vi "MatlabfileReader.vi"(8 "error in (no error)":errorcluster, 11 "Positions file":path) -> (0 "error out":errorcluster, 1 "Focus":dbl[](array[numeric]), 2 "Y":dbl[](array[numeric]), 3 "X":dbl[](array[numeric]), 5 "Time":dbl[](array[numeric]))   [LabVIEW 2012]
uses:
  <vilib>/Utility/file.llb/Read From Spreadsheet File (DBL).vi
  <vilib>/Analysis/NI_AALBase.lvlib
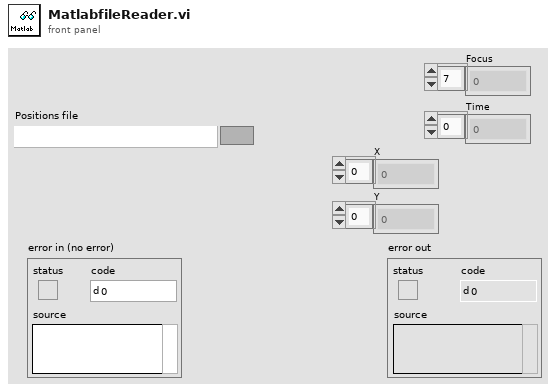
[diagram p1: front panel]
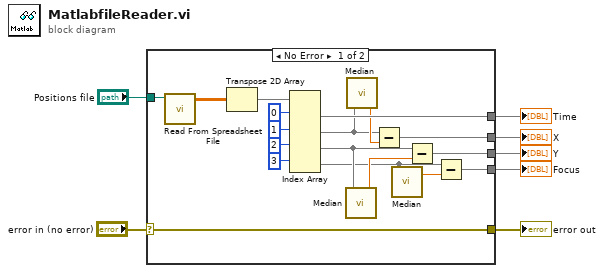
[diagram p0: block diagram]
diagram:
  n1 = case shown="No Error" "error in (no error)" {
    selector: "error in (no error)" -> [w20 w26]
    tunnel: [w20 w26] -> w6
    tunnel: "Positions file" -> [w25 _]
    tunnel: [w21 _] -> w4
    tunnel: [w14 _] -> w2
    tunnel: [w12 _] -> w3
    tunnel: [w13 _] -> w1
    frame No Error {
      n2 = call-poly <vilib>:"Read From Spreadsheet File.vi"("file path (dialog if empty)"=w25) -> ("all rows"=w24:dbl[][])  [unwired: 6 in, 4 out]
      n3 = Transpose 2D Array(2D array=w24) -> (transposed array=w19:dbl[][])
      n4 = Index Array(array=w19, index (row) #1=0 ("index (row)"), index (row) #2=1 ("index (row)"), index (row) #3=2 ("index (row)"), index (row) #4=3 ("index (row)")) -> (element #1=w21:dbl[], element #2=w15:dbl[], element #3=w11:dbl[], element #4=w9:dbl[])  [unwired: 4 in]
      n5 = call <vilib>:"Median.vi"("X"=w11) -> ("median"=w10:dbl)  [unwired: 1 out]
      n6 = call <vilib>:"Median.vi"("X"=w15) -> ("median"=w16:dbl)  [unwired: 1 out]
      n7 = Subtract(x=w15, y=w16) -> (x-y=w14:dbl[])
      n8 = call <vilib>:"Median.vi"("X"=w9) -> ("median"=w8:dbl)  [unwired: 1 out]
      n9 = Subtract(x=w11, y=w10) -> (x-y=w13:dbl[])
      n10 = Subtract(x=w9, y=w8) -> (x-y=w12:dbl[])
    }
    frame Error {
    }
  }
  "error out" <- w6
  "Focus" <- w3
  "Time" <- w4
  "X" <- w2
  "Y" <- w1
